vi "AlliGator Get DAQ & Metadata.vi"(8 "Error In":errorcluster) -> (0 "Error Out":errorcluster, 1 "Metadata":string, 3 "DAQ Parameters":T1)   [LabVIEW 2021, in "AlliGator HDF5.lvlib"]
doc: "Gets <B>DAQ Parameters</b> and <B>Metadata</B> string from internal data storage."
uses:
  AlliGator HDF5.lvlib
  Phasor/Phasor Fluorescence Lifetime Parameters v3.ctl
  AlliGator HDF5 File Dataset Parameters Steps.ctl
  AlliGator Variables List.ctl
  AlliGator Baseline Subtraction Method.ctl
  AlliGator Gates to Skip.ctl
  AlliGator Settings List.ctl
  AlliGator Globals.vi
  Variant/Variant to Data/Variant to DBL.vi
  Variant/Variant to Data/Variant to U32.vi
  Variant/Variant to Data/Variant to Boolean.vi
  Variant/Variant to Data/Variant to Path.vi
  Variant/Variant to Data/Variant to I32.vi
  Variant/Variant to Data/Variant to String.vi
  AlliGator Globals, Variables & Constants.lvlib
  Variant/Variant to Data/Variant to Data.lvlib
  AlliGator Settings.lvlib
  AlliGator Decay Preprocessing.lvlib
  AlliGator Decay Analysis.lvlib
  Phasor/Phasor.lvlib
  Variant/Variant.lvlib
panel:
  # "see the AlliGator License on the block diagram (Ctrl+E or Window:Show Block Diagram)"
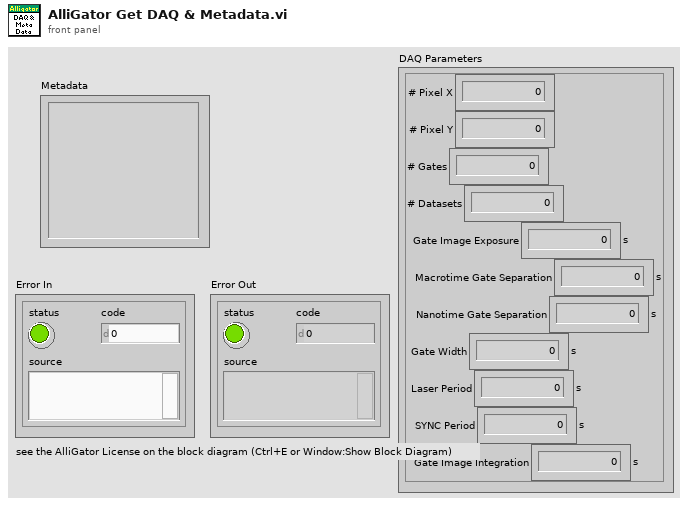
[diagram p1: front panel]
types:
  T1 = typedef "Phasor.lvlib/Phasor Fluorescence Lifetime Parameters v3.ctl" = cluster{"# Pixel X":i32, "# Pixel Y":i32, "# Gates":i32, "# Datasets":i32, "Gate Image Exposure":dbl[unit], "Macrotime Gate Separation":dbl[unit], "Nanotime Gate Separation":dbl[unit], "Gate Width":dbl[unit], "Laser Period":dbl[unit], "SYNC Period":dbl[unit], "Gate Image Integration":dbl[unit]}
  T2 = typedef "AlliGator HDF5.lvlib/AlliGator HDF5 File Dataset Parameters Steps.ctl" = enum16{"metadata: Background File Subtraction", "metadata: Background Subtraction", "metadata: Dataset Accumulation", "metadata: Gate Choice", "metadata: Corrections", "Dataset Information", "DAQ Parameters"}
  T3 = typedef "AlliGator Globals, Variables & Constants.lvlib/AlliGator Variables List.ctl" = enum16{"---- GUI ----", "Initialization Status", "State Indicators Refnum", "Original AlliGator Menu Items", "Current Action Loop State", "Script in progress", "Playback", "Loop Playback", "Search ROI Used", "Search ROI", "Decay Graph Max Legend Size", "Intensity Graph Max Legend Size", "Decay Statistics Graph Max Legend Size", "Phasor Graph Max Legend Size", "Phasor Ratio Graph Max Legend Size", "Lifetime Graph Max Legend Size", "---- Files ----", "Export Dataset Frames as Individual Files", "Show Batch Export Help Balloons", "Frames in Dataset", "ptu File Frame Start Indices", "Current Frame in Dataset", "Current Frame Timestamp", "------ Python Plugins ------", "Python Plugins Information", "Python Session", "Valid Python Session?", "---- Source Image ----", "Dataset Loaded", "Dataset Metadata", "Dataset Channel", "Dataset Data Description", "Background Dataset Metadata", "Background Dataset Channel", "Background Dataset Data Description", "Background File Subtraction", "Background File Path", "Background File Pile-up Correction", "Background File Pixel Well Capacity", "Background File Scaling Factor", "Source Image ROIs", "Current Source Image ROI", "Source Image ROI Event Refnum", "X_Source Image Display Range", "X_Source Image Palette Information", "Source Image Palette List", "Source Image Scale", "Current Dataset Load Settings", "Source Image:ROI Overlay Color", "---- Image Profile Window ----", "Image Profile:Overlay ROI in Source Image", "Image Profile Window Event Refnum", "Image Profile:IntensityType", "Image Profile:Intensity Average Type", "Image Profile:Intensity-weighted SDV", "Image Profile:Box Profile Type", "Image Profile Window Open", "Image Profile:Plotted Fit Parameter", "X_Type of Displayed Image", "X_Time Gate Slider", "Dataset Path", "Source Image Overlay to Erase", "Is Displayed Image Accumulated", "White Light Image Modified", "Mask Image Modified", "Macrotime Gate Separation", "------ Phasor Graph -------", "Phasor Graph:Show Line", "---- Phasor Plot ---", "Phasor Plot Parameters Changed", "FLI Dataset Modified since last Phasor Plot Calculation", "Phasor Harmonics Data", "Selected Phasor Harmonics", "Phasor Harmonic Manager Event Refnum", "Phasor Plot ROIs", "Current Phasor Plot ROI", "Phasor Plot ROI Event Refnum", "Phasor Plot Image Reference Points", "Phasor Plot Computed", "Phasor Plot Palette Information", "Phasor Plot Palette List", "Phasor Ratio Palette Information", "Phasor Ratio Palette List", "Phasor Image Scale", "Phasor Plot Image Overlay to Erase", "Phasor Plot Image Elements to Update", "Current Phasor Plot Calculation Parameters", "Current Phasor Calibration Options", "Reset Cumulated Phasor Plot", "Phasor Ratio Reference 1", "Phasor Ratio Lifetime Reference 1", "Phasor Ratio Reference 1 Frequency", "Phasor Ratio Reference 2", "Phasor Ratio Lifetime Reference 2", "Phasor Ratio Reference 2 Frequency", "---- Decay Analysis ----", "Number of Selected Decays to Fit", "LS Fit Results", "LAR Fit Results", "BS Fit Results", "Last Decay Max - Min", "Best Fit Parameters", "Best Fit Parameter Names", "Actual Size X", "Actual Size Y", "Binning X", "Binning Y", "Actual # Gates", "Dataset Number", "Gates to...", "Gates Skipped", "Gates to keep", "Gate Step", "Gate Separation", "Reversed Gates", "Pile-up Correction", "Pixel Well Capacity", "Background Subtracted", "Background Subtraction Method", "Background Definition Range", "Background File (deprecated)", "Number of Dataset Accumulated", "Array of Accumulated Dataset Paths", "Do Averaged Datasets", "Destination File Path", "Process Plot Target", "Use 1/D as Phasor Frequency", "---- Decay Fit Parameter Map -----", "Decay Fit Parameter Map Palette Information", "Decay Fit Parameter Map Palette List", "Local Decay Graph Window Event Refnum", "------- Local Decay Window ---------", "Use normalized IRF for convolution", "----- Miscellaneous ----", "Skippable Dialog Windows Status"}
  T4 = cluster{"Min Gate":dbl[unit], "Max Gate":dbl[unit]}
  T5 = typedef "AlliGator Decay Analysis.lvlib/AlliGator Decay Preprocessing.lvlib/AlliGator Baseline Subtraction Method.ctl" = enum16{"Mean", "Min", "Square Gated Single-Exponential", "File", "Constant"}
  T6 = typedef "AlliGator Decay Analysis.lvlib/AlliGator Gates to Skip.ctl" = cluster{"Start":u32, "End":u32}
  T7 = typedef "AlliGator Settings.lvlib/AlliGator Settings List.ctl" = enum16{"GUI:Visible Settings Tab", "GUI:Last Run Version", "Source Image:Use Image Histogram for Contrast", "Source Image:Low Count Pixels Rejection Options", "Source Image:High Count Pixels Rejection Options", "Source Image:Use Image Brightness", "Source Image:Blend Overlay with Image Background", "Source Image:Use Fixed ROI Diameter", "Source Image:ROI Diameter", "Source Image:ROI Center Color", "Source Image:Peak Threshold", "Source Image:Intensity Threshold", "Source Image:Image Binning Options", "Source Image:Image Smoothing Options", "Source Image:Image Histogram Active", "Source Image:Invert Binary Mask", "Source Image:Hot Pixel Removal", "Source Image:Overlay Analyzed ROI Center", "Source Image:Auto-Adjust Contrast", "Source Image:Histogram Lower Percentile", "Source Image:Histogram Upper Percentile", "Source Image:Save Source Image", "Source Image:Scale Bar Options", "Source Image:Image Resolution (Pixel Size)", "Source Image:Flatfield Correction", "Data Information:Gate Width", "Data Information:Nanotime Gate Separation", "Data Information:Macrotime Gate Separation", "Data Information:Gate Step", "Data Information:# Gates", "Data Information:Gate Image Exposure", "Data Information:Gate Image Integration", "Data Information:Gates to Skip", "Data Information:Gates to Keep", "Data Information:Define Gates to", "Data Information:Channel Name", "Data Information:Available Channel Names", "Data Information:Channel Arithmetic", "Data Information:Background File Subtraction", "Data Information:Background File", "Data Information:Background Scaling Factor", "Data Information:Background Pile-up Correction", "Data Information:Background Pixel Well Capacity", "Data Information:Laser Period", "Data Information:SYNC Period", "Data Information:Pile-up Correction", "Data Information:Pixel Well Capacity", "Data Information:Dataset Scaling Factor", "Fluorescence Decay_Decay Pre-Processing:Reverse Gates", "Fluorescence Decay_Decay Pre-Processing:Verbose Decay Pre-Processing", "Fluorescence Decay_Decay Pre-Processing:Use Decay Pre-Processing", "Fluorescence Decay_Decay Pre-Processing:Background Subtraction", "Fluorescence Decay_Decay Pre-Processing:Background Definition Range", "Fluorescence Decay_Decay Pre-Processing:Baseline Subtraction Method", "Fluorescence Decay_Decay Pre-Processing:Operations Order", "Fluorescence Decay_Decay Pre-Processing:Smoothing Parameter", "Fluorescence Decay_Decay Pre-Processing:Shift Decay", "Fluorescence Decay_Decay Pre-Processing:Decay Shift Parameters", "Fluorescence Decay_Decay Pre-Processing:Fold Decay", "Fluorescence Decay_Decay Pre-Processing:# Folds", "Fluorescence Decay_Decay Pre-Processing:1-Normalize Decay", "Fluorescence Decay_Decay Pre-Processing:[0-1]-Normalize Decay", "Fluorescence Decay_Decay Pre-Processing:Smoothen Decay", "Fluorescence Decay_Decay Pre-Processing:Extrapolate Decay", "Fluorescence Decay_Decay Pre-Processing:Use Periodicity", "Fluorescence Decay_Decay Pre-Processing:Use Cursors", "Fluorescence Decay_Decay Pre-Processing:Tail Fraction", "Fluorescence Decay_Decay Pre-Processing:Head Fraction", "Fluorescence Decay_Decay Pre-Processing:Additional Points", "Fluorescence Decay_Decay Pre-Processing:Straighten Decay", "Fluorescence Decay_Decay Pre-Processing:Constant Background", "Fluorescence Decay_Decay Pre-Processing:Pixel-Normalize Decay", "Fluorescence Decay_Advanced Analysis:Extract IRF instead of Decay", "Fluorescence Decay_Advanced Analysis:IRF Extraction Options", "Fluorescence Decay_Advanced Analysis:IRF Optimization Options", "Fluorescence Decay_Advanced Analysis:Square Pulse Options", "Fluorescence Decay_Advanced Analysis:IRF Order", "Fluorescence Decay_Advanced Analysis:IRF Time Constants", "Fluorescence Decay_Advanced Analysis:Wavelet Analysis Options", "Fluorescence Decay_Advanced Analysis:Average Lifetime Options", "Fluorescence Decay_Fit Options:Fit Options", "Fluorescence Decay_Fit Options:Use Legacy Fitting Approach", "Fluorescence Decay_Fit Options:Use Data Information Laser Period", "Fluorescence Decay_Fit Parameters:Displayed Fit Parameters", "Fluorescence Decay_Fit Parameters:Fit Parameter Constraints", "Fluorescence Decay_Fit Parameters:Export Tabulated Results", "Fluorescence Decay_Fit Parameters:MLE Baseline Offset Type", "Fluorescence Decay_Fit Parameters:MLE Baseline Offset", "Fluorescence Decay_Fit Parameters:Guess Parameter Names", "Fluorescence Decay_Fit Parameters:Guess Parameter Values", "Fluorescence Decay_Fit Parameters:Guess Parameters Options", "Fluorescence Decay_Styles:Show Last Decay Only", "Fluorescence Decay_Styles:Decay Graph Color Array", "Fluorescence Decay:Decay Graph Active", "Fluorescence Decay Statistics:Min Peak Value", "Fluorescence Decay Statistics:Reject Low Decay Peak Pixels", "Fluorescence Decay Statistics:Reject High Decay Peak Pixels", "Fluorescence Decay Statistics:Max Peak Value", "Time Traces:Use File Timestamp", "Time Traces:Time Step", "Time Traces:Use Intensity Correction File", "Time Traces:Intensity Correction File", "Phasor Plot:Phasor Plot Smoothing Options", "Phasor Plot:Phasor Plot Size", "Phasor Plot:Phasor Plot Graphics Options", "Phasor Plot:Cumulative Phasor Plot", "Phasor Plot:Use Phasor Brightness", "Phasor Plot:Blend Overlay with Phasor Background", "Phasor Plot:Save Phasor Plot", "Phasor Plot:Show References", "Phasor Plot:Phasor Ratio Decay Range", "Phasor Plot:Exponential Fading", "Phasor Plot:Phasor Ratio Reference Colors", "Phasor Plot:Reference Radius", "Phasor Plot:Show Color Map Vertices", "Phasor Plot:Phasor Plot Active", "Phasor Plot:Phasor Ratio Color Map Type", "Phasor Plot:Phasor Ratio Color Map", "Phasor Plot:Phasor Ratio Display Range", "Phasor Plot:Selected Image ROI(s)", "Phasor Plot:All Image ROIs", "Phasor Plot:Selected Phasor Plot ROI(s)", "Phasor Plot:All Phasor Plot ROIs", "Phasor Plot:Phasor Ratio Color-Coded Quantity", "Phasor Plot:Store Phasor Harmonics", "Phasor Plot:Draw Reference Segment", "Phasor Plot:User-Defined Quantity", "Phasor Graph:Phasor Frequency", "Phasor Graph:Phasor Ratio Type", "Phasor Graph:Pixel-level Phasor Computation", "Phasor Graph:Save Phasor Graph", "Phasor Graph:Phasor Graph Active", "Phasor Graph:Phasor SDV Options", "Phasor Calibration:Use Backup Calibration if needed", "Phasor Graph:Define Shortest Lifetime as", "Phasor Calibration:Backup Calibration Type", "Phasor Calibration:Calibration Type", "Phasor Calibration:Calibration Lifetime", "Phasor Calibration:Calibration Map Algorithm", "Single-Exponential Phasor Locus (SEPL):Gate Parameters", "Single-Exponential Phasor Locus (SEPL):User-defined Gate", "Single-Exponential Phasor Locus (SEPL):User-defined IRF", "Single-Exponential Phasor Locus (SEPL):Phasor Parameters", "Single-Exponential Phasor Locus (SEPL):Decay & IRF Parameters", "Single-Exponential Phasor Locus (SEPL):Display Parameters", "Lifetime Analysis:Decay Analysis Parameters", "Lifetime Analysis:Lifetime Map Active", "Plugins:Python Settings", "Miscellaneous:Verbose Mode", "Miscellaneous:Beep after Script", "Miscellaneous:Saved Image File Format", "Miscellaneous:Exported Gate Image Settings", "Miscellaneous:Include Loading in Timing", "Miscellaneous:Verbose Settings Mode", "Miscellaneous:Histogram Options", "Miscellaneous:Beep on Error", "Miscellaneous:# Logical Processors Used", "Miscellaneous:ROI Description Max Characters", "Miscellaneous:Verbose Error Mode", "Miscellaneous:Transparent Mask Color"}
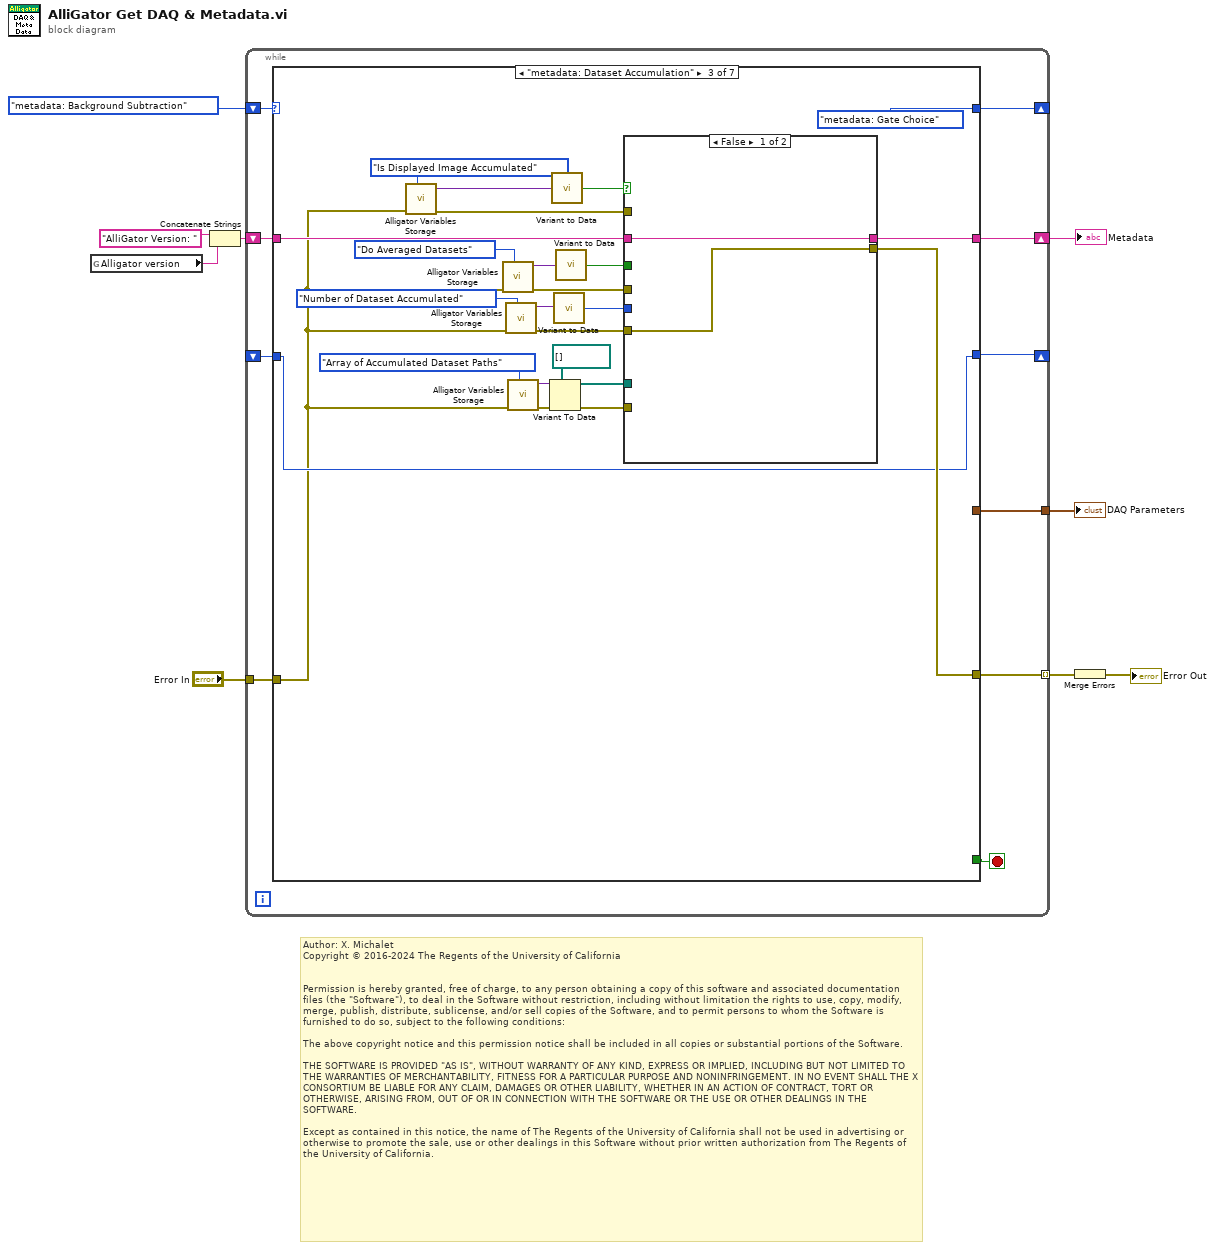
[diagram p0: block diagram]
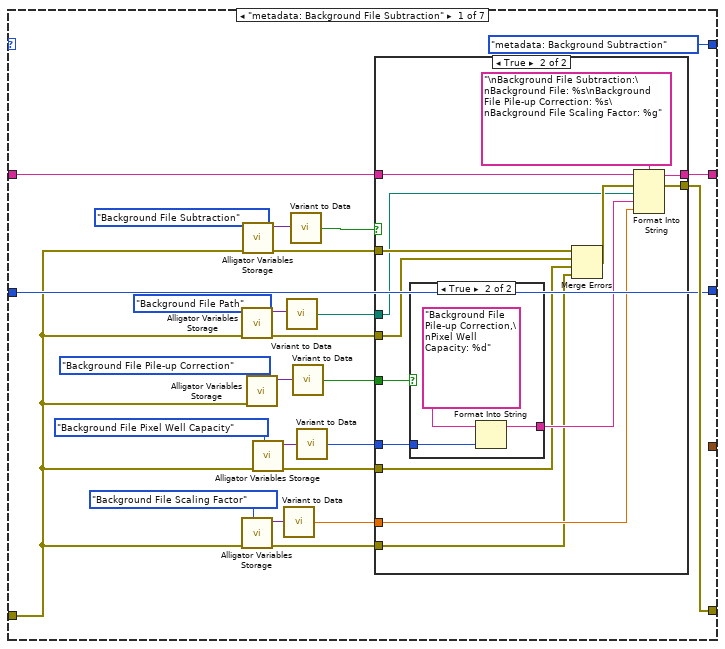
[diagram p2: hidden frame]
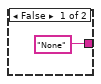
[diagram p4: hidden frame]
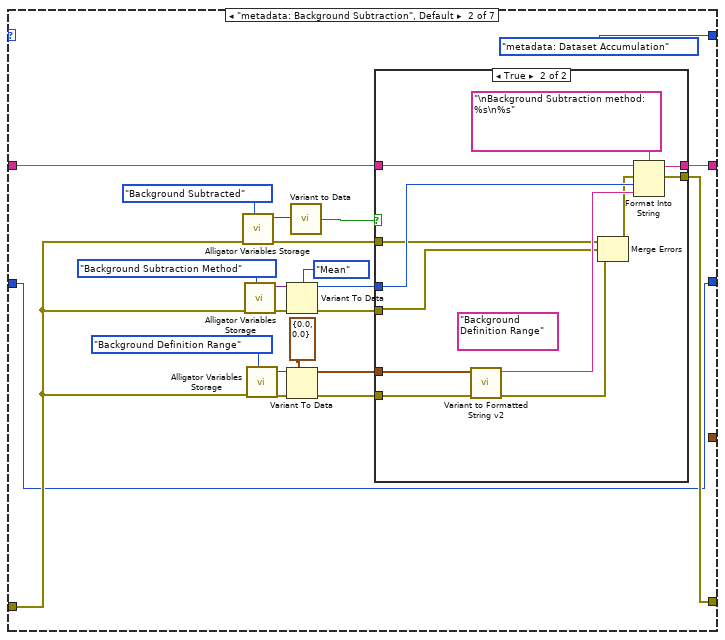
[diagram p5: hidden frame]
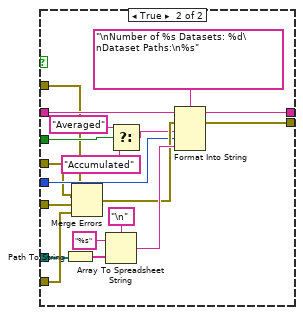
[diagram p7: hidden frame]
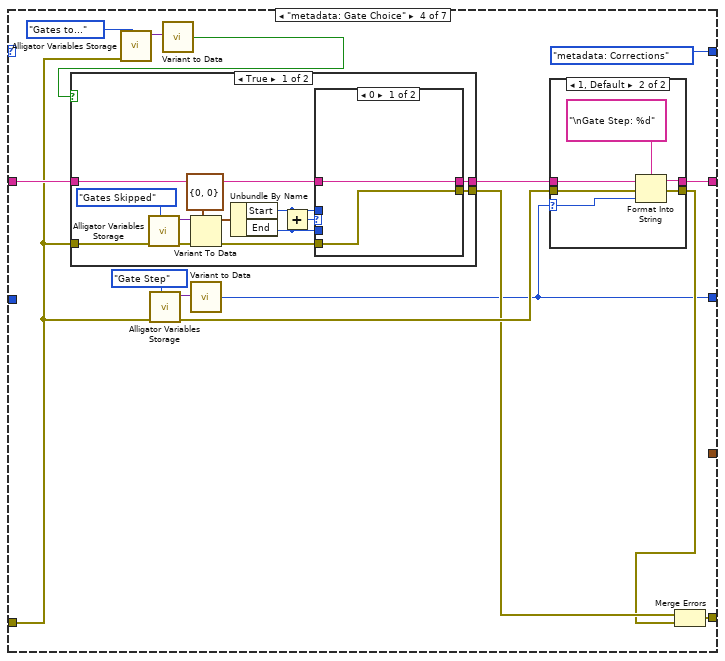
[diagram p8: hidden frame]
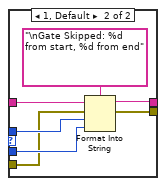
[diagram p9: hidden frame]
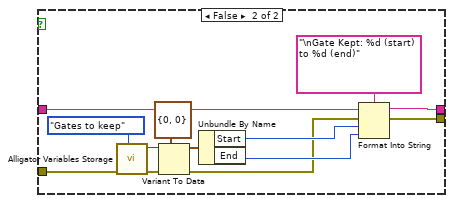
[diagram p10: hidden frame]
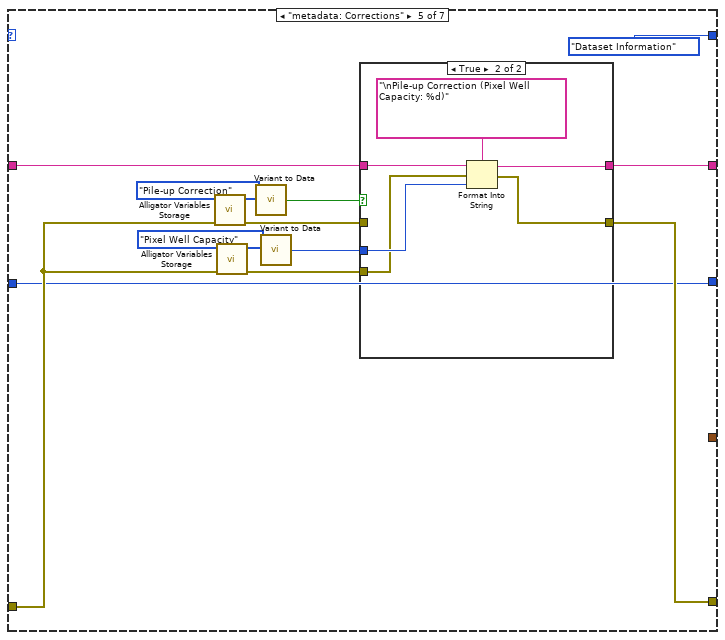
[diagram p12: hidden frame]
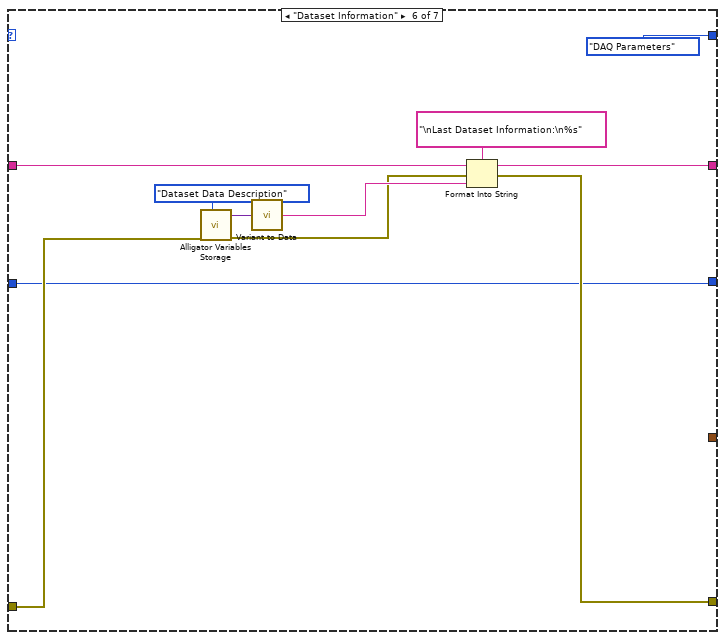
[diagram p14: hidden frame]
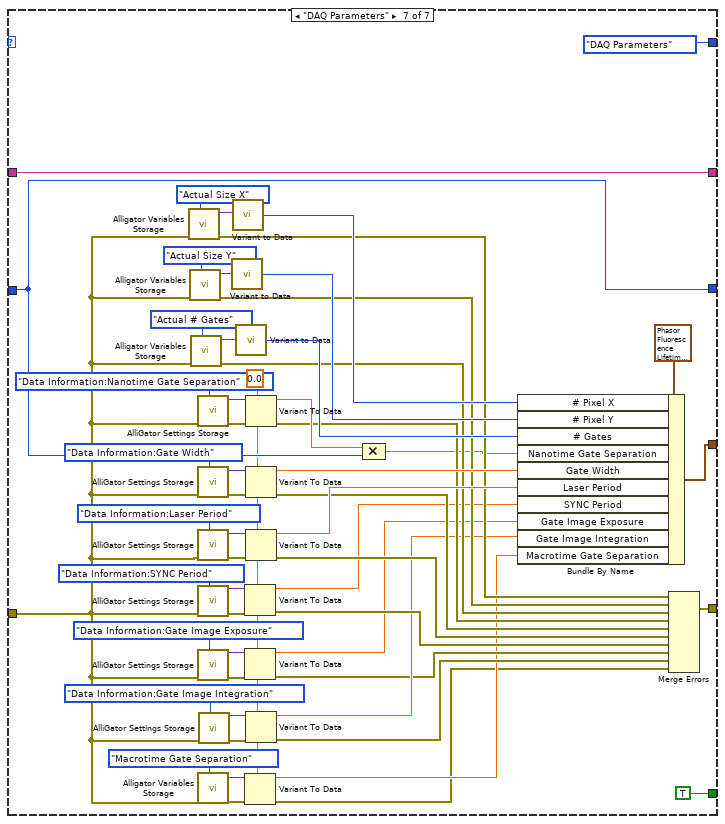
[diagram p15: hidden frame]
diagram:
  # "Author: X. Michalet\nCopyright © 2016-2024 The Regents of the University of California\n \n\nPermission is hereby granted, free of charge, to any person obtaining a copy of this software and associated documentation files (the \"Software\"), to deal in the Software without restriction, including without limitation the rights to use, copy, modify, merge, publish, distribute, sublicense, and/or sell copies of the Software, and to permit persons to whom the Software is furnished to do so, subject to the following conditions:\n\nThe above copyright notice and this permission notice shall be included in all copies or substantial portions of the Software.\n\nTHE SOFTWARE IS PROVIDED \"AS IS\", WITHOUT WARRANTY OF ANY KIND, EXPRESS OR IMPLIED, INCLUDING BUT NOT LIMITED TO THE WARRANTIES OF MERCHANTABILITY, FITNESS FOR A PARTICULAR PURPOSE AND NONINFRINGEMENT. IN NO EVENT SHALL THE X CONSORTIUM BE LIABLE FOR ANY CLAIM, DAMAGES OR OTHER LIABILITY, WHETHER IN AN ACTION OF CONTRACT, TORT OR OTHERWISE, ARISING FROM, OUT OF OR IN CONNECTION WITH THE SOFTWARE OR THE USE OR OTHER DEALINGS IN THE SOFTWARE.\n\nExcept as contained in this notice, the name of The Regents of the University of California shall not be used in advertising or otherwise to promote the sale, use or other dealings in this Software without prior written authorization from The Regents of the University of California."
  n1 = global read "AlliGator Globals.vi" "Alligator version"() -> (w4:string)
  n2 = Concatenate Strings("AlliGator Version: " ("string"), w4) -> (w5:string)
  n3 = while {
    tunnel: "Error In" -> [w18]
    shift-right: [w15] -> w6
    shift-left: w5 -> [w16]
    tunnel: [w14] -> w3 mode=indexing
    tunnel: [w13] -> w1
    shift-right: [w12] -> _
    shift-left: AlliGator_HDF5_File_Dataset_Parameters_Steps."metadata: Background Subtraction" -> [w19]
    shift-right: [w11] -> _
    shift-left: _ -> [w10]
    stop <- w17 stop-if-true
    n4 = case shown="\"metadata: Dataset Accumulation\"" w19 {
      tunnel: w18 -> [w29 w75 w104 w148 w215 w234 w240]
      tunnel: [_ _ _ _ _ _ TRUE] -> w17
      tunnel: [w34 w69 w112 w159 w206 w228 w269] -> w14
      tunnel: w16 -> [w39 w81 w120 w158 w214 w233 w270]
      tunnel: [w38 w80 w119 w155 w213 w232 w270] -> w15
      tunnel: [_ _ _ _ _ _ w271] -> w13
      tunnel: [AlliGator_HDF5_File_Dataset_Parameters_Steps."metadata: Background Subtraction" AlliGator_HDF5_File_Dataset_Parameters_Steps."metadata: Dataset Accumulation" AlliGator_HDF5_File_Dataset_Parameters_Steps."metadata: Gate Choice" AlliGator_HDF5_File_Dataset_Parameters_Steps."metadata: Corrections" AlliGator_HDF5_File_Dataset_Parameters_Steps."Dataset Information" AlliGator_HDF5_File_Dataset_Parameters_Steps."DAQ Parameters" AlliGator_HDF5_File_Dataset_Parameters_Steps."DAQ Parameters"] -> w12
      tunnel: [w31 w65 w106 w150 w204 w226 w255] -> w11
      tunnel: w10 -> [w31 w65 w106 _ w204 w226 w255]
      frame "metadata: Background File Subtraction" {
        n5 = call "Alligator Variables Storage.vi"("AlliGator Variable"=AlliGator_Variables_List."Background File Path" ("Alligator Variable"), "Error In"=w29) -> ("Error Out"=w26:errorcluster, "Data out"=w28:variant)  [unwired: 7 in, 1 out]
        n6 = call "Alligator Variables Storage.vi"("AlliGator Variable"=AlliGator_Variables_List."Background File Scaling Factor" ("Alligator Variable"), "Error In"=w29) -> ("Error Out"=w20:errorcluster, "Data out"=w24:variant)  [unwired: 7 in, 1 out]
        n7 = call "Alligator Variables Storage.vi"("AlliGator Variable"=AlliGator_Variables_List."Background File Subtraction" ("Alligator Variable"), "Error In"=w29) -> ("Error Out"=w33:errorcluster, "Data out"=w41:variant)  [unwired: 7 in, 1 out]
        n8 = call "Alligator Variables Storage.vi"("AlliGator Variable"=AlliGator_Variables_List."Background File Pile-up Correction" ("Alligator Variable"), "Error In"=w29) -> ("Data out"=w25:variant)  [unwired: 7 in, 2 out]
        n9 = call "Alligator Variables Storage.vi"("AlliGator Variable"=AlliGator_Variables_List."Background File Pixel Well Capacity" ("Alligator Variable"), "Error In"=w29) -> ("Error Out"=w21:errorcluster, "Data out"=w36:variant)  [unwired: 7 in, 1 out]
        n10 = call-poly "Variant to Data.vi"("Variant"=w24) -> ("Value"=w22:dbl)  [unwired: 8 in]
        n11 = call-poly "Variant to Data.vi"("Variant"=w28) -> ("Path"=w27:path)  [unwired: 8 in]
        n12 = call-poly "Variant to Data.vi"("Variant"=w41) -> ("Value"=w40:bool)  [unwired: 8 in]
        n13 = call-poly "Variant to Data.vi"("Variant"=w25) -> ("Value"=w23:bool)  [unwired: 8 in]
        n14 = call-poly "Variant to Data.vi"("Variant"=w36) -> ("Value"=w35:u32)  [unwired: 8 in]
        n15 = case shown="True" w40 {
          tunnel: w39 -> [w46 w60]
          tunnel: [w46 w58] -> w38
          tunnel: w35 -> [_ w51]
          tunnel: [w45 w57] -> w34
          tunnel: w33 -> [w45 w55]
          tunnel: w27 -> [_ w54]
          tunnel: w26 -> [_ w53]
          tunnel: w23 -> [_ w52]
          tunnel: w22 -> [_ w49]
          tunnel: w21 -> [_ w48]
          tunnel: w20 -> [_ w47]
          frame False {
          }
          frame True {
            n16 = case shown="True" w52 {
              tunnel: w51 -> [_ w63]
              tunnel: ["None" ("input 2") w64] -> w50
              frame False {
              }
              frame True {
                n17 = Format Into String(initial string="Background File Pile-up Correction,\nPixel Well Capacity: %d", w63) -> (resulting string=w64:string)  [unwired: 2 in, 1 out]
              }
            }
            n18 = Merge Errors(w55, w53, w48, w47) -> (w56:errorcluster)
            n19 = Format Into String(format string="\nBackground File Subtraction:\nBackground File: %s\nBackground File Pile-up Correction: %s\nBackground File Scaling Factor: %g", initial string=w60, error in=w56, w54, w50, w49) -> (resulting string=w58:string, error out=w57:errorcluster)
          }
        }
      }
      frame "metadata: Background Subtraction", Default {
        n20 = call "Alligator Variables Storage.vi"("AlliGator Variable"=AlliGator_Variables_List."Background Subtracted" ("Alligator Variable"), "Error In"=w75) -> ("Error Out"=w68:errorcluster, "Data out"=w83:variant)  [unwired: 7 in, 1 out]
        n21 = call "Alligator Variables Storage.vi"("AlliGator Variable"=AlliGator_Variables_List."Background Subtraction Method" ("Alligator Variable"), "Error In"=w75) -> ("Error Out"=w79:errorcluster, "Data out"=w78:variant)  [unwired: 7 in, 1 out]
        n22 = call "Alligator Variables Storage.vi"("AlliGator Variable"=AlliGator_Variables_List."Background Definition Range" ("Alligator Variable"), "Error In"=w75) -> ("Error Out"=w74:errorcluster, "Data out"=w73:variant)  [unwired: 7 in, 1 out]
        n23 = Variant To Data(error in=w79, type=AlliGator_Baseline_Subtraction_Method."Mean" ("Baseline Subtraction Method"), Variant=w78) -> (data=w76:T5, error out=w67:errorcluster)
        n24 = Variant To Data(error in=w74, type=T4 {"Min Gate"=0.0, "Max Gate"=0.0}, Variant=w73) -> (data=w71:T4, error out=w70:errorcluster)
        n25 = call-poly "Variant to Data.vi"("Variant"=w83) -> ("Value"=w82:bool)  [unwired: 8 in]
        n26 = case shown="True" w82 {
          tunnel: w81 -> [w88 w100]
          tunnel: [w88 w97] -> w80
          tunnel: w76 -> [_ w98]
          tunnel: w71 -> [_ w96]
          tunnel: w70 -> [_ w95]
          tunnel: [w87 w92] -> w69
          tunnel: w68 -> [w87 w90]
          tunnel: w67 -> [_ w89]
          frame False {
          }
          frame True {
            (unwired) "Background Definition Range" ("Label")
            n27 = call "Variant to Formatted String v2.vi"("error in (no error)"=w95, "Anything"=w96) -> ("error out"=w93:errorcluster, "String"=w94:string)  [unwired: 8 in]
            n28 = Merge Errors(w90, w89, w93) -> (w91:errorcluster)
            n29 = Format Into String(format string="\nBackground Subtraction method: %s\n%s", initial string=w100, error in=w91, w98, w94) -> (resulting string=w97:string, error out=w92:errorcluster)
          }
        }
      }
      frame "metadata: Dataset Accumulation" {
        n30 = call "Alligator Variables Storage.vi"("AlliGator Variable"=AlliGator_Variables_List."Is Displayed Image Accumulated" ("Alligator Variable"), "Error In"=w104) -> ("Error Out"=w101:errorcluster, "Data out"=w103:variant)  [unwired: 7 in, 1 out]
        n31 = call "Alligator Variables Storage.vi"("AlliGator Variable"=AlliGator_Variables_List."Do Averaged Datasets" ("Alligator Variable"), "Error In"=w104) -> ("Error Out"=w107:errorcluster, "Data out"=w109:variant)  [unwired: 7 in, 1 out]
        n32 = call "Alligator Variables Storage.vi"("AlliGator Variable"=AlliGator_Variables_List."Number of Dataset Accumulated" ("Alligator Variable"), "Error In"=w104) -> ("Error Out"=w114:errorcluster, "Data out"=w122:variant)  [unwired: 7 in, 1 out]
        n33 = call "Alligator Variables Storage.vi"("AlliGator Variable"=AlliGator_Variables_List."Array of Accumulated Dataset Paths" ("Alligator Variable"), "Error In"=w104) -> ("Error Out"=w118:errorcluster, "Data out"=w117:variant)  [unwired: 7 in, 1 out]
        n34 = Variant To Data(error in=w118, type=path[] [], Variant=w117) -> (data=w116:path[], error out=w113:errorcluster)
        n35 = call-poly "Variant to Data.vi"("Variant"=w103) -> ("Value"=w102:bool)  [unwired: 8 in]
        n36 = call-poly "Variant to Data.vi"("Variant"=w122) -> ("Value"=w121:i32)  [unwired: 8 in]
        n37 = call-poly "Variant to Data.vi"("Variant"=w109) -> ("Value"=w108:bool)  [unwired: 8 in]
        n38 = case shown="False" w102 {
          tunnel: w120 -> [w126 w145]
          tunnel: [w126 w143] -> w119
          tunnel: w116 -> [_ w140]
          tunnel: w114 -> [w125 w142]
          tunnel: w113 -> [_ w141]
          tunnel: [w125 w135] -> w112
          tunnel: w108 -> [_ w132]
          tunnel: w107 -> [_ w128]
          tunnel: w121 -> [_ w133]
          tunnel: w101 -> [_ w127]
          frame False {
          }
          frame True {
            n39 = Path To String(path=w140) -> (string=w139:string[])
            n40 = Merge Errors(w127, w128, w142, w141) -> (w136:errorcluster)
            n41 = Array To Spreadsheet String(delimiter (Tab)="\n", array=w139, 3:"%s" ("format string")) -> (spreadsheet string=w137:string)
            n42 = Select(t="Averaged" ("string"), s=w132, f="Accumulated" ("string")) -> (s? t:f=w129:string)
            n43 = Format Into String(format string="\nNumber of %s Datasets: %d\nDataset Paths:\n%s", initial string=w145, error in=w136, w129, w133, w137) -> (resulting string=w143:string, error out=w135:errorcluster)
          }
        }
      }
      frame "metadata: Gate Choice" {
        n44 = call "Alligator Variables Storage.vi"("AlliGator Variable"=AlliGator_Variables_List."Gates to..." ("Alligator Variable"), "Error In"=w148) -> ("Data out"=w147:variant)  [unwired: 7 in, 2 out]
        n45 = call "Alligator Variables Storage.vi"("AlliGator Variable"=AlliGator_Variables_List."Gate Step" ("Alligator Variable"), "Error In"=w148) -> ("Error Out"=w154:errorcluster, "Data out"=w157:variant)  [unwired: 7 in, 1 out]
        n46 = call-poly "Variant to Data.vi"("Variant"=w147) -> ("Value"=w146:bool)  [unwired: 8 in]
        n47 = case shown="True" w146 {
          tunnel: w158 -> [w172 w194]
          tunnel: [w164 w187] -> w156
          tunnel: [w162 w185] -> w153
          tunnel: w148 -> [w161 w184]
          frame True {
            n48 = call "Alligator Variables Storage.vi"("AlliGator Variable"=AlliGator_Variables_List."Gates Skipped" ("Alligator Variable"), "Error In"=w161) -> ("Error Out"=w171:errorcluster, "Data out"=w170:variant)  [unwired: 7 in, 1 out]
            n49 = Variant To Data(error in=w171, type=T6 {"Start"=0, "End"=0} ("Gates to Skip"), Variant=w170) -> (data=w168:T6, error out=w163:errorcluster)
            n50 = Unbundle By Name(w168) -> ("Start"=w166:u32, "End"=w165:u32)
            n51 = Add(x=w166, y=w165) -> (x+y=w167:u32)
            n52 = case shown="0" w167 {
              tunnel: w172 -> [w175 w182]
              tunnel: [w175 w180] -> w164
              tunnel: w166 -> [_ w179]
              tunnel: w165 -> [_ w178]
              tunnel: w163 -> [w174 w177]
              tunnel: [w174 w176] -> w162
              frame 0 {
              }
              frame 1, Default {
                n53 = Format Into String(format string="\nGate Skipped: %d from start, %d from end", initial string=w182, error in=w177, w179, w178) -> (resulting string=w180:string, error out=w176:errorcluster)
              }
            }
          }
          frame False {
            n54 = call "Alligator Variables Storage.vi"("AlliGator Variable"=AlliGator_Variables_List."Gates to keep" ("Alligator Variable"), "Error In"=w184) -> ("Error Out"=w193:errorcluster, "Data out"=w192:variant)  [unwired: 7 in, 1 out]
            n55 = Variant To Data(error in=w193, type=T6 {"Start"=0, "End"=0} ("Gates to Skip"), Variant=w192) -> (data=w190:T6, error out=w186:errorcluster)
            n56 = Unbundle By Name(w190) -> ("Start"=w189:u32, "End"=w188:u32)
            n57 = Format Into String(format string="\nGate Kept: %d (start) to %d (end)", initial string=w194, error in=w186, w189, w188) -> (resulting string=w187:string, error out=w185:errorcluster)
          }
        }
        n58 = call-poly "Variant to Data.vi"("Variant"=w157) -> ("Value"=w150:u32)  [unwired: 8 in]
        n59 = case shown="1, Default" w150 {
          selector: w150 -> [_ w198]
          tunnel: [w197 w202] -> w155
          tunnel: w156 -> [w197 w201]
          tunnel: w154 -> [w196 w200]
          tunnel: [w196 w199] -> w152
          frame 0 {
          }
          frame 1, Default {
            n60 = Format Into String(format string="\nGate Step: %d", initial string=w201, error in=w200, w198) -> (resulting string=w202:string, error out=w199:errorcluster)
          }
        }
        n61 = Merge Errors(w153, w152) -> (w159:errorcluster)
      }
      frame "metadata: Corrections" {
        n62 = call "Alligator Variables Storage.vi"("AlliGator Variable"=AlliGator_Variables_List."Pile-up Correction" ("Alligator Variable"), "Error In"=w215) -> ("Error Out"=w207:errorcluster, "Data out"=w212:variant)  [unwired: 7 in, 1 out]
        n63 = call "Alligator Variables Storage.vi"("AlliGator Variable"=AlliGator_Variables_List."Pixel Well Capacity" ("Alligator Variable"), "Error In"=w215) -> ("Error Out"=w208:errorcluster, "Data out"=w210:variant)  [unwired: 7 in, 1 out]
        n64 = call-poly "Variant to Data.vi"("Variant"=w212) -> ("Value"=w211:bool)  [unwired: 8 in]
        n65 = call-poly "Variant to Data.vi"("Variant"=w210) -> ("Value"=w209:u32)  [unwired: 8 in]
        n66 = case shown="True" w211 {
          tunnel: w214 -> [w219 w225]
          tunnel: [w219 w223] -> w213
          tunnel: w209 -> [_ w222]
          tunnel: w208 -> [_ w221]
          tunnel: w207 -> [w218 _]
          tunnel: [w218 w220] -> w206
          frame False {
          }
          frame True {
            n67 = Format Into String(format string="\nPile-up Correction (Pixel Well Capacity: %d)", initial string=w225, error in=w221, w222) -> (resulting string=w223:string, error out=w220:errorcluster)
          }
        }
      }
      frame "Dataset Information" {
        n68 = call "Alligator Variables Storage.vi"("AlliGator Variable"=AlliGator_Variables_List."Dataset Data Description" ("Alligator Variable"), "Error In"=w234) -> ("Error Out"=w229:errorcluster, "Data out"=w235:variant)  [unwired: 7 in, 1 out]
        n69 = call-poly "Variant to Data.vi"("Variant"=w235) -> ("String"=w230:string)  [unwired: 8 in]
        n70 = Format Into String(format string="\nLast Dataset Information:\n%s", initial string=w233, error in=w229, w230) -> (resulting string=w232:string, error out=w228:errorcluster)
      }
      frame "DAQ Parameters" {
        w243 = dbl[unit] 0.0 ("Gate Duration")
        n71 = call "Alligator Variables Storage.vi"("AlliGator Variable"=AlliGator_Variables_List."Actual Size X" ("Alligator Variable"), "Error In"=w240) -> ("Error Out"=w268:errorcluster, "Data out"=w289:variant)  [unwired: 7 in, 1 out]
        n72 = call "Alligator Variables Storage.vi"("AlliGator Variable"=AlliGator_Variables_List."Actual Size Y" ("Alligator Variable"), "Error In"=w240) -> ("Error Out"=w267:errorcluster, "Data out"=w288:variant)  [unwired: 7 in, 1 out]
        n73 = call "Alligator Variables Storage.vi"("AlliGator Variable"=AlliGator_Variables_List."Actual # Gates" ("Alligator Variable"), "Error In"=w240) -> ("Error Out"=w266:errorcluster, "Data out"=w292:variant)  [unwired: 7 in, 1 out]
        n74 = call "AlliGator Settings Storage.vi"("AlliGator Settings List"=AlliGator_Settings_List."Data Information:Nanotime Gate Separation", "Error In"=w240) -> ("Error Out"=w287:errorcluster, "Variant Data out"=w285:variant)  [unwired: 8 in]
        n75 = call "AlliGator Settings Storage.vi"("AlliGator Settings List"=AlliGator_Settings_List."Data Information:Gate Width", "Error In"=w240) -> ("Error Out"=w280:errorcluster, "Variant Data out"=w279:variant)  [unwired: 8 in]
        n76 = call "AlliGator Settings Storage.vi"("AlliGator Settings List"=AlliGator_Settings_List."Data Information:Laser Period", "Error In"=w240) -> ("Error Out"=w282:errorcluster, "Variant Data out"=w283:variant)  [unwired: 8 in]
        n77 = call "AlliGator Settings Storage.vi"("AlliGator Settings List"=AlliGator_Settings_List."Data Information:SYNC Period", "Error In"=w240) -> ("Error Out"=w260:errorcluster, "Variant Data out"=w259:variant)  [unwired: 8 in]
        n78 = call "AlliGator Settings Storage.vi"("AlliGator Settings List"=AlliGator_Settings_List."Data Information:Gate Image Exposure", "Error In"=w240) -> ("Error Out"=w253:errorcluster, "Variant Data out"=w254:variant)  [unwired: 8 in]
        n79 = call "Alligator Variables Storage.vi"("AlliGator Variable"=AlliGator_Variables_List."Macrotime Gate Separation" ("Alligator Variable"), "Error In"=w240) -> ("Error Out"=w239:errorcluster, "Data out"=w238:variant)  [unwired: 7 in, 1 out]
        n80 = call "AlliGator Settings Storage.vi"("AlliGator Settings List"=AlliGator_Settings_List."Data Information:Gate Image Integration", "Error In"=w240) -> ("Error Out"=w250:errorcluster, "Variant Data out"=w249:variant)  [unwired: 8 in]
        n81 = call-poly "Variant to Data.vi"("Variant"=w288) -> ("Value"=w291:i32)  [unwired: 8 in]
        n82 = call-poly "Variant to Data.vi"("Variant"=w289) -> ("Value"=w290:i32)  [unwired: 8 in]
        n83 = call-poly "Variant to Data.vi"("Variant"=w292) -> ("Value"=w293:i32)  [unwired: 8 in]
        n84 = Variant To Data(error in=w260, type=w243, Variant=w259) -> (data=w257:dbl[unit], error out=w256:errorcluster)
        n85 = Variant To Data(error in=w253, type=w243, Variant=w254) -> (data=w251:dbl[unit], error out=w246:errorcluster)
        n86 = Variant To Data(error in=w239, type=w243, Variant=w238) -> (data=w242:dbl[unit], error out=w241:errorcluster)
        n87 = Variant To Data(error in=w287, type=w243, Variant=w285) -> (data=w286:dbl[unit], error out=w265:errorcluster)
        n88 = Variant To Data(error in=w280, type=w243, Variant=w279) -> (data=w281:dbl[unit], error out=w264:errorcluster)
        n89 = Variant To Data(error in=w282, type=w243, Variant=w283) -> (data=w284:dbl[unit], error out=w263:errorcluster)
        n90 = Variant To Data(error in=w250, type=w243, Variant=w249) -> (data=w247:dbl[unit], error out=w245:errorcluster)
        n91 = Compound Arithmetic op=MULTIPLY(w286, w255) -> (w261:dbl[unit])
        n92 = Bundle By Name(cluster=T1 {"# Pixel X"=0, "# Pixel Y"=0, "# Gates"=0, "# Datasets"=0, "Gate Image Exposure"=0.0, "Macrotime Gate Separation"=0.0, "Nanotime Gate Separation"=0.0, "Gate Width"=0.0, "Laser Period"=0.0, "SYNC Period"=0.0, "Gate Image Integration"=0.0} ("DAQ Parameters"), "# Pixel X"=w290, "# Pixel Y"=w291, "# Gates"=w293, "Nanotime Gate Separation"=w261, "Gate Width"=w281, "Laser Period"=w284, "SYNC Period"=w257, "Gate Image Exposure"=w251, "Gate Image Integration"=w247, "Macrotime Gate Separation"=w242) -> (w271:T1)
        n93 = Merge Errors(w268, w267, w266, w265, w264, w263, w256, w246, w245, w241) -> (w269:errorcluster)
      }
    }
  }
  "Metadata" <- w6
  "DAQ Parameters" <- w1
  n94 = Merge Errors(w3) -> (→"Error Out":errorcluster)
